vi "Average Cycle Bandwidth.vi"(10 "Decimation":u64=1, 11 "Buffer":refnum<class "Buffer.lvclass">) -> (3 "average cycle bandwidth":dbl format="%.0g bytes")   [LabVIEW 2017]
uses:
  Classes/Buffer/Buffer.lvclass
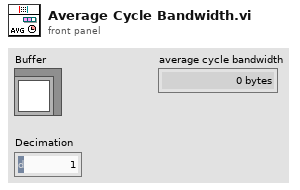
[diagram p1: front panel]
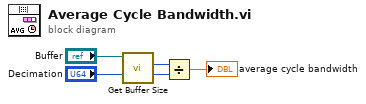
[diagram p0: block diagram]
diagram:
  n1 = call "Get Buffer Size.vi"("Buffer in"="Buffer") -> ("buffer size"=w1:u64)  [unwired: 9 in, 1 out]
  n2 = Divide(x=w1, y="Decimation") -> (x/y=→"average cycle bandwidth":dbl)
